vi "Release Rabbits.vi"(8 "error in (no error)":errorcluster, 11 "Rabbit Squad in":refnum<class "Rabbit Squad.lvclass">) -> (0 "error out":errorcluster, 3 "Rabbit Squad out":refnum<class "Rabbit Squad.lvclass">)   [LabVIEW 2014, in "Rabbit Squad.lvclass"]
uses:
  Rabbit Squad.lvclass
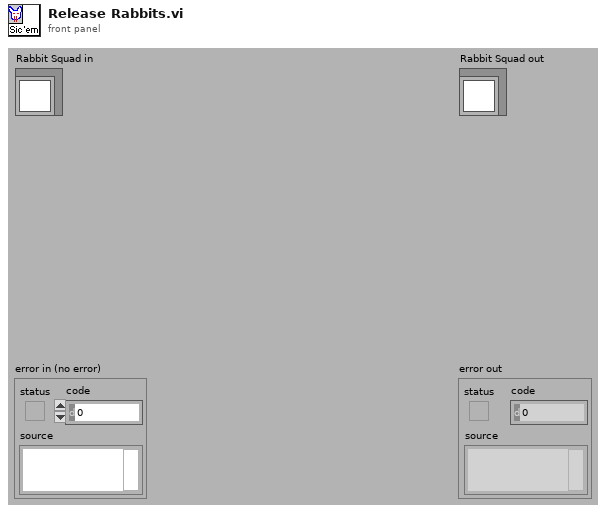
[diagram p1: front panel]
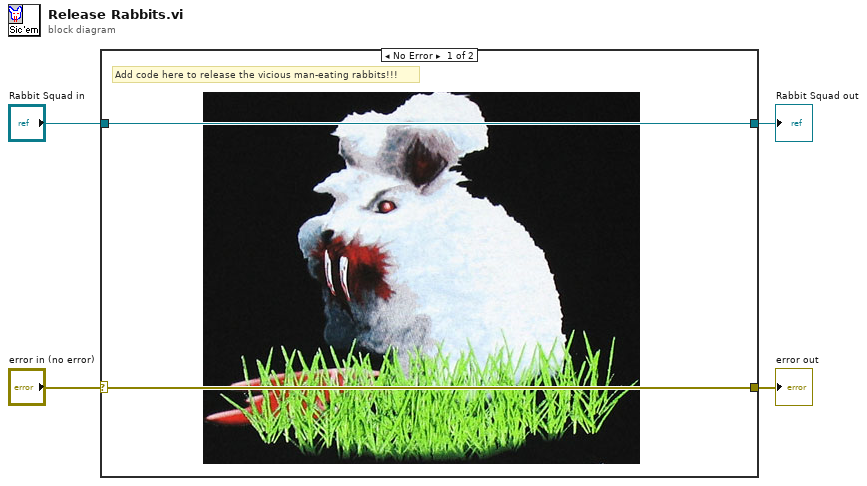
[diagram p0: block diagram]
diagram:
  n1 = case shown="No Error" "error in (no error)" {
    selector: "error in (no error)" -> [w5 w8]
    tunnel: [w5 w8] -> w3
    tunnel: [w6 w7] -> w1
    tunnel: "Rabbit Squad in" -> [w6 w7]
    frame No Error {
      # "Add code here to release the vicious man-eating rabbits!!!"
    }
    frame Error {
    }
  }
  "error out" <- w3
  "Rabbit Squad out" <- w1
